vi "Pre Launch Init.vi"(11 "Tracer-V in":refnum<class "Tracer-V.lvclass">) -> (0 "error out":errorcluster, 3 "Tracer-V out":refnum<class "Tracer-V.lvclass">)   [LabVIEW 2013, in "Tracer-V.lvclass"]
doc: "(<B>Filename</B>: Actor Framework.lvlib:Actor.lvclass:Pre Launch Init.vi)\n\nDefines behavior that occurs after the Launch Actor method is invoked but before the actor's Actor Core method begins running.\n\nThe Pre Launch Init method is guaranteed to finish before the Launch Actor method returns to its caller and before the actor itself receives any messages. Any references that the Pre Launch Init method obtains are guaranteed to have the same lifetime as the actor itself. Any errors that the Pre Launch Init method returns will abort the launch.\n\nBy default, this method does nothing. A descendant class may override it to define behavior."
uses:
  Tracer-V.lvclass
  Tracer-V.lvclass/Tracer-V.ctl
  Logical Systems/TraceMessage/Trace.lvclass
  Logical Systems/Tracer/Tracer.lvclass
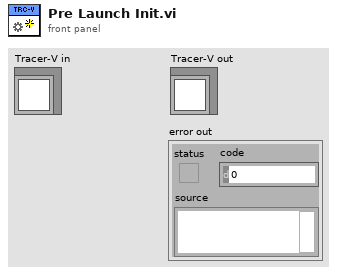
[diagram p1: front panel]
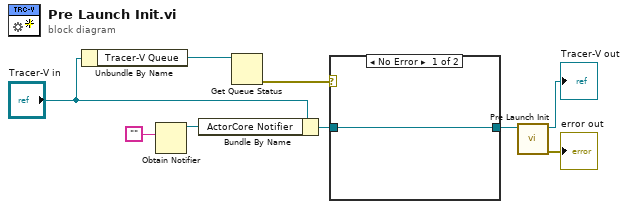
[diagram p0: block diagram]
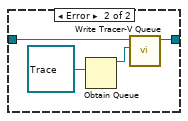
[diagram p2: hidden frame]
diagram:
  n1 = Unbundle By Name("Tracer-V in") -> ("Tracer-V Queue"=w7:refnum<queue>)
  n2 = Obtain Notifier(notification data type="") -> (notifier out=w1:refnum<notifier>)  [unwired: 3 in, 2 out]
  n3 = Bundle By Name(cluster="Tracer-V in", "ActorCore Notifier"=w1) -> (w2:refnum<class "Tracer-V.lvclass">)
  n4 = Get Queue Status(queue=w7) -> (error out=w6:errorcluster)  [unwired: 2 in, 7 out]
  n5 = case shown="No Error" w6 {
    tunnel: w2 -> [w10 w14]
    tunnel: [w10 w13] -> w4
    frame No Error {
    }
    frame Error {
      n6 = Obtain Queue(element data type=refnum<class "Trace.lvclass"> refnum ("Trace.lvclass")) -> (queue out=w11:refnum<queue>)  [unwired: 4 in, 2 out]
      n7 = call-dynamic "Write Tracer-V Queue.vi"("TraceMessage Queue"=w11, "Tracer-V in"=w14) -> ("Tracer-V out"=w13:refnum<class "Tracer-V.lvclass">)  [unwired: 8 in, 1 out]
    }
  }
  n8 = call-parent "Pre Launch Init.vi"("Actor in"=w4) -> ("error out"=→"error out":errorcluster, "Actor out"=→"Tracer-V out":refnum<class "Tracer-V.lvclass">)  [unwired: 9 in]
